vi "IMAQ color table presets.vi"(11 "Color table":T1=enum."enhance low") -> (2 "Make new one cancelled":bool, 3 "Array":cluster{"R":u8, "G":u8, "B":u8}[](array[cluster]))   [LabVIEW 2020]
uses:
  color tables/image color table presets.ctl
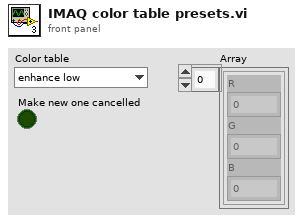
[diagram p1: front panel]
types:
  T1 = typedef "image color table presets.ctl" = enum16{"Greyscale", "Binary", "Gradient", "Rainbow", "Temperature", "enhance low", "blue yellow red", "BYR enhance low", "white blue yellow", "BWR enhance low", "make a new one"}
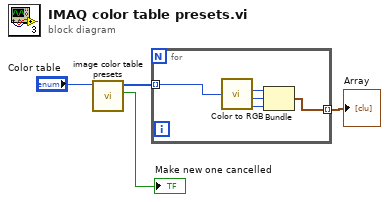
[diagram p0: block diagram]
diagram:
  n1 = call "image color table presets.vi"("Color table"="Color table") -> ("Make new one cancelled"=→"Make new one cancelled":bool, "white to yellow color table"=w4:u32[])  [unwired: 9 in]
  n2 = for {
    tunnel: w4 -> [w6] mode=indexing
    tunnel: [w5] -> w3 mode=indexing
    n3 = call <vilib>:"Color to RGB.vi"("Color"=w6) -> ("R"=w9:u8, "G"=w8:u8, "B"=w7:u8)  [unwired: 1 out]
    n4 = Bundle("R"=w9, "G"=w8, "B"=w7) -> (w5:cluster{"R":u8, "G":u8, "B":u8})  [unwired: 1 in]
  }
  "Array" <- w3
